vi "Extract LSS Styles.vi"(8 "Error in":errorcluster, 11 "File Without Comments":string) -> (0 "Error out":errorcluster, 3 "LSS Styles":T1[](array[typedef]))   [LabVIEW 2019, in "LSS.lvlib"]
doc: "This VI takes the input Style Sheet and outputs a cluster of information containing the information from the style sheet parsed into a useable format. If the style sheet does not follow the standard conventions this will return an error indicating what is wrong with the style sheet.\n\nInputs:\n<b>File Without Comments</b> - Style Sheet with the comment sections already removed. This VI will return an error if the input is blank.\n<b>Error In</b> - Error in terminal\n\nOutputs:\n<b>Style Sheet</b> - Array of clusters containing the information from the style sheet.\n<b>Error Out</b> - Error out terminal"
uses:
  LSS.lvlib
  Controls/Style.ctl
  <vilib>/Utility/error.llb/Error Cluster From Error Code.vi
  <vilib>/regexp/Match Regular Expression.xnode
  <vilib>/ErrorRing/Error Ring.xnode
panel:
  out "Error Text":string
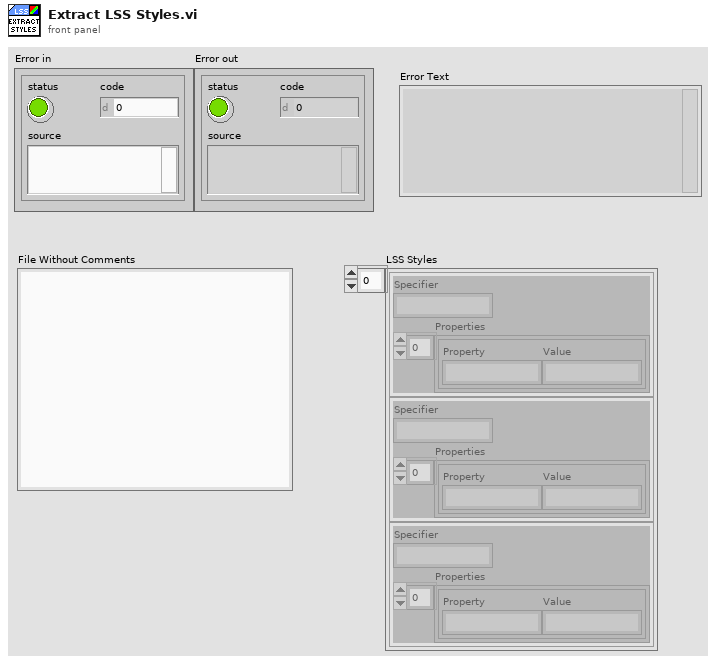
[diagram p1: front panel]
types:
  T1 = typedef "LSS.lvlib/Style.ctl" = cluster{"Specifier":string, "Properties":cluster{"Property":string, "Value":string}[]}
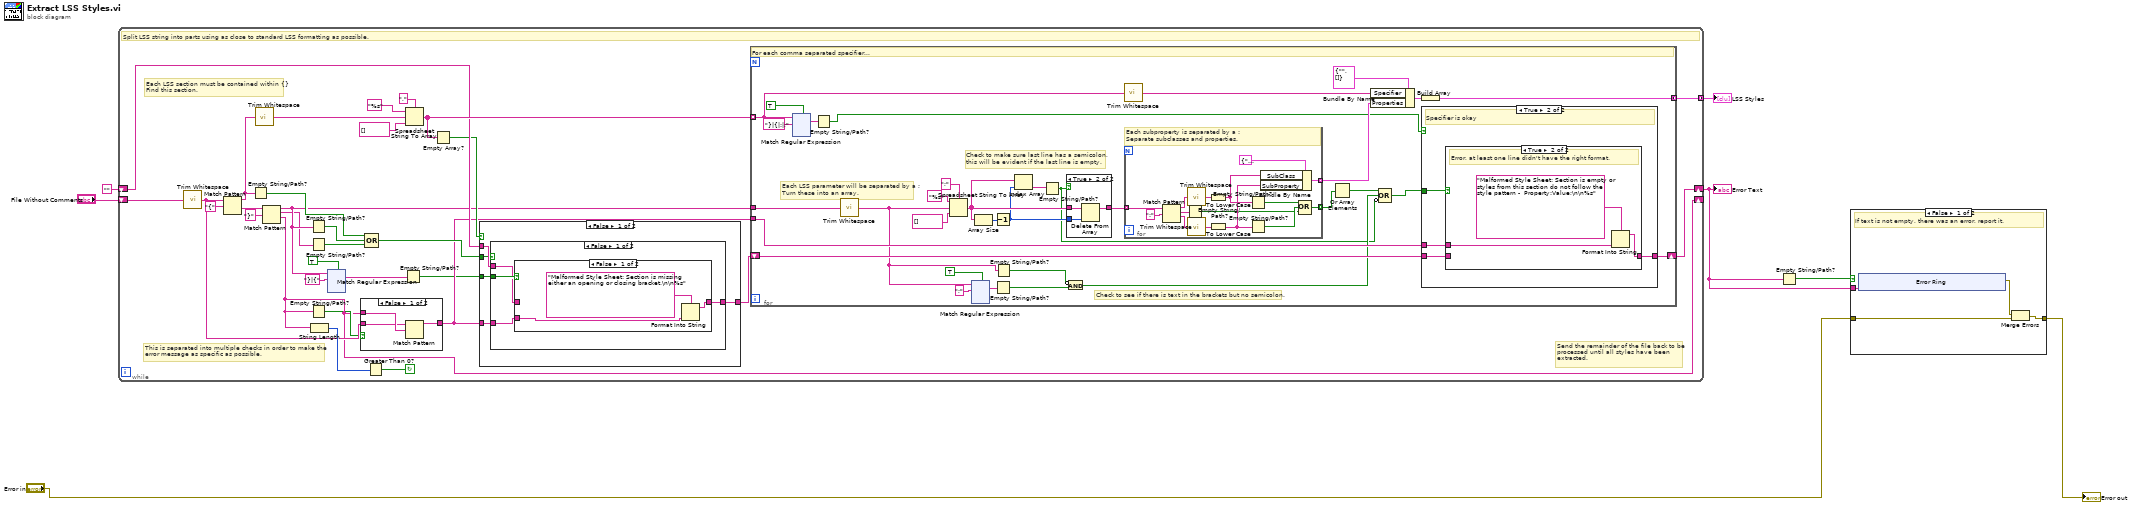
[diagram p0: block diagram]
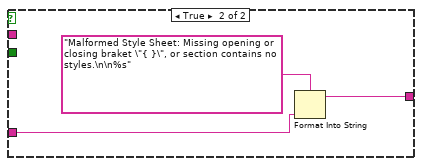
[diagram p5: hidden frame]
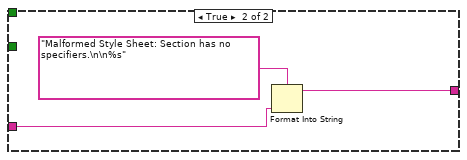
[diagram p6: hidden frame]
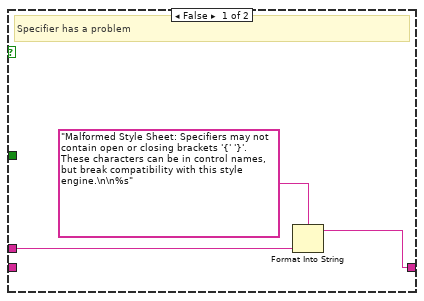
[diagram p8: hidden frame]
diagram:
  n1 = while {
    shift-right: [w18] -> _
    shift-left: "File Without Comments" -> [w21]
    tunnel: [w33] -> w6 mode=concatenating
    shift-right: [w16] -> w1
    shift-left: "" -> [w24]
    stop <- w35 continue-if-true
    # "This is separated into multiple checks in order to make the\nerror message as specific as possible."
    # "Send the remainder of the file back to be\nprocessed until all styles have been\nextracted."
    # "Each LSS section must be contained within {}\nFind this section."
    # "Split LSS string into parts using as close to standard LSS formatting as possible."
    n2 = call <vilib>:"Trim Whitespace.vi"("string"=w21) -> ("trimmed string"=w20:string)  [unwired: 1 in]
    n3 = Match Pattern(string=w20, regular expression="{" ("search string/char (-)")) -> (before substring=w22:string, after substring=w34:string)  [unwired: 1 in, 2 out]
    n4 = Empty String/Path?(string/path=w22) -> (empty?=w26:bool)
    n5 = call <vilib>:"Trim Whitespace.vi"("string"=w22) -> ("trimmed string"=w29:string)  [unwired: 1 in]
    n6 = Match Pattern(string=w34, regular expression="}" ("search string/char (-)")) -> (before substring=w12:string, match substring=w9:string, after substring=w18:string)  [unwired: 1 in, 1 out]
    n7 = Empty String/Path?(string/path=w12) -> (empty?=w27:bool)
    n8 = Empty String/Path?(string/path=w9) -> (empty?=w8:bool)
    n9 = Empty String/Path?(string/path=w18) -> (empty?=w19:bool)
    n10 = String Length(string=w18) -> (length=w36:i32)
    n11 = xnode "Match Regular Expression"("input string"=w12, "regular expression"="}|{", "multiline? (F)"=TRUE) -> ("whole match"=w11:string)  [unwired: 3 in, 4 out]
    n12 = case shown="False" w19 {
      tunnel: w18 -> [w155 _]
      tunnel: [w154 w156] -> w15
      tunnel: w20 -> [w153 w156]
      frame False {
        n13 = Match Pattern(string=w153, regular expression=w155) -> (before substring=w154:string)  [unwired: 1 in, 3 out]
      }
      frame True {
      }
    }
    n14 = Compound Arithmetic op=OR(w26, w27, w8) -> (w25:bool)
    n15 = Greater Than 0?(x=w36) -> (x > 0?=w35:bool)
    n16 = Empty String/Path?(string/path=w11) -> (empty?=w10:bool)
    n17 = Spreadsheet String To Array(delimiter (Tab)=",", format string="%s", spreadsheet string=w29, array type (2D Dbl)=string[] [] ("appended array")) -> (array=w28:string[])
    n18 = Empty Array?(array=w28) -> (empty?=w23:bool)
    n19 = case shown="False" w23 {
      tunnel: w25 -> [w158 _]
      tunnel: w24 -> [w161 _]
      tunnel: [w160 w173] -> w17
      tunnel: w15 -> [w159 w174]
      tunnel: w10 -> [w157 _]
      frame False {
        n20 = case shown="False" w158 {
          tunnel: w161 -> [w164 _]
          tunnel: [w163 w171] -> w160
          tunnel: w159 -> [w162 w170]
          tunnel: w157 -> [w165 _]
          frame False {
            n21 = case shown="False" w165 {
              tunnel: w164 -> [_ w169]
              tunnel: [w166 w169] -> w163
              tunnel: w162 -> [w167 _]
              frame False {
                n22 = Format Into String(format string="Malformed Style Sheet: Section is missing either an opening or closing bracket.\n\n%s" ("source"), w167) -> (resulting string=w166:string)  [unwired: 2 in, 1 out]
              }
              frame True {
              }
            }
          }
          frame True {
            n23 = Format Into String(format string="Malformed Style Sheet: Missing opening or closing braket \"{ }\", or section contains no styles.\n\n%s" ("source"), w170) -> (resulting string=w171:string)  [unwired: 2 in, 1 out]
          }
        }
      }
      frame True {
        n24 = Format Into String(format string="Malformed Style Sheet: Section has no specifiers.\n\n%s" ("source"), w174) -> (resulting string=w173:string)  [unwired: 2 in, 1 out]
      }
    }
    n25 = for {
      tunnel: w12 -> [w208]
      tunnel: [w202] -> w33 mode=concatenating
      tunnel: w28 -> [w188] mode=indexing
      shift-right: [w196] -> w16
      shift-left: w17 -> [w197]
      tunnel: w15 -> [w195]
      # "Check to make sure last line has a semicolon,\nthis will be evident if the last line is empty."
      # "Check to see if there is text in the brackets but no semicolon."
      # "Each LSS parameter will be separated by a ;\nTurn these into an array."
      # "For each comma separated specifier..."
      n26 = xnode "Match Regular Expression"("input string"=w188, "regular expression"="}|{|:|;", "multiline? (F)"=TRUE) -> ("whole match"=w191:string)  [unwired: 3 in, 4 out]
      n27 = Empty String/Path?(string/path=w191) -> (empty?=w187:bool)
      n28 = call <vilib>:"Trim Whitespace.vi"("string"=w208) -> ("trimmed string"=w181:string)  [unwired: 1 in]
      n29 = Spreadsheet String To Array(delimiter (Tab)=";", format string="%s", spreadsheet string=w181, array type (2D Dbl)=string[] [] ("appended array")) -> (array=w179:string[])
      n30 = xnode "Match Regular Expression"("input string"=w181, "regular expression"=";", "multiline? (F)"=TRUE) -> ("whole match"=w184:string)  [unwired: 3 in, 4 out]
      n31 = Array Size(array=w179) -> (size(s)=w201:i32)
      n32 = Decrement(x=w201) -> (x-1=w178:i32)
      n33 = Empty String/Path?(string/path=w184) -> (empty?=w183:bool)
      n34 = Empty String/Path?(string/path=w181) -> (empty?=w182:bool)
      n35 = Index Array(array=w179, index=w178) -> (element=w177:string)
      n36 = Empty String/Path?(string/path=w177) -> (empty?=w176:bool)
      n37 = case shown="True" w176 {
        tunnel: w178 -> [_ w212]
        tunnel: [w209 w211] -> w200
        tunnel: w179 -> [w209 w210]
        frame False {
        }
        frame True {
          n38 = Delete From Array(array=w210, index=w212) -> (array with subset deleted=w211:string[])  [unwired: 1 in, 1 out]
        }
      }
      n39 = Compound Arithmetic op=AND(invert w182, w183) -> (w180:bool)
      n40 = call <vilib>:"Trim Whitespace.vi"("string"=w188) -> ("trimmed string"=w198:string)  [unwired: 1 in]
      n41 = for {
        tunnel: w200 -> [w466] mode=indexing
        tunnel: [w465] -> w199 mode=indexing
        tunnel: [w452] -> w192 mode=indexing
        # "Each subproperty is separated by a :\nSeparate subclasses and properties."
        n42 = Match Pattern(string=w466, regular expression=":") -> (before substring=w463:string, match substring=w454:string, after substring=w462:string)  [unwired: 1 in, 1 out]
        n43 = Empty String/Path?(string/path=w454) -> (empty?=w453:bool)
        n44 = call <vilib>:"Trim Whitespace.vi"("string"=w463) -> ("trimmed string"=w460:string)  [unwired: 1 in]
        n45 = call <vilib>:"Trim Whitespace.vi"("string"=w462) -> ("trimmed string"=w459:string)  [unwired: 1 in]
        n46 = To Lower Case(string=w460) -> (all lower case string=w458:string)
        n47 = To Lower Case(string=w459) -> (all lower case string=w457:string)
        n48 = Empty String/Path?(string/path=w458) -> (empty?=w456:bool)
        n49 = Empty String/Path?(string/path=w457) -> (empty?=w455:bool)
        n50 = Bundle By Name(cluster=cluster{"SubClass":string, "SubProperty":string} {"SubClass"="", "SubProperty"=""} ("Property"), "SubClass"=w458, "SubProperty"=w457) -> (w465:cluster{"SubClass":string, "SubProperty":string})
        n51 = Compound Arithmetic op=OR(w456, w455, w453) -> (w452:bool)
      }
      n52 = Or Array Elements(Boolean array=w192) -> (logical OR=w193:bool)
      n53 = Bundle By Name(cluster=T1 {"Specifier"="", "Properties"=[]}, "Specifier"=w198, "Properties"=w199) -> (w203:T1)
      n54 = Compound Arithmetic op=OR(w193, w180, invert w176) -> (w194:bool)
      n55 = Build Array(w203) -> (w202:T1[])
      n56 = case shown="True" w187 {
        tunnel: w197 -> [_ w333]
        tunnel: [w327 w332] -> w196
        tunnel: w195 -> [w328 w331]
        tunnel: w194 -> [_ w330]
        frame False {
          # "Specifier has a problem"
          n57 = Format Into String(format string="Malformed Style Sheet: Specifiers may not contain open or closing brackets '{' '}'.  These characters can be in control names, but break compatibility with this style engine.\n\n%s" ("source"), w328) -> (resulting string=w327:string)  [unwired: 2 in, 1 out]
        }
        frame True {
          # "Specifier is okay"
          n58 = case shown="True" w330 {
            tunnel: w333 -> [w334 _]
            tunnel: [w334 w335] -> w332
            tunnel: w331 -> [_ w336]
            frame False {
              # "No error."
            }
            frame True {
              # "Error, at least one line didn't have the right format."
              n59 = Format Into String(format string="Malformed Style Sheet: Section is empty or styles from this section do not follow the style pattern -  Property:Value;\n\n%s" ("source"), w336) -> (resulting string=w335:string)  [unwired: 2 in, 1 out]
            }
          }
        }
      }
    }
  }
  "LSS Styles" <- w6
  "Error Text" <- w1
  n60 = Empty String/Path?(string/path=w1) -> (empty?=w4:bool)
  n61 = case shown="False" w4 {
    tunnel: "Error in" -> [w469 w478]
    tunnel: [w470 w478] -> w2
    tunnel: w1 -> [w468 _]
    frame False {
      # "If text is not empty, there was an error, report it."
      n62 = xnode "Error Ring"("parameter 0"=w468) -> ("error out"=w467:errorcluster)
      n63 = Merge Errors(w467, w469) -> (w470:errorcluster)
    }
    frame True {
      # "Text is empty, no LSS errors."
    }
  }
  "Error out" <- w2
